vi "TMC.vi"() -> (0 "Position":u32, 1 "Encoder Readout":dbl format="%.3f")   [LabVIEW 2019]
uses:
  TMC Global.vi
panel:
  in  "stop":bool
  in  "Move Up":bool
  out "Soft Down Limit":bool
  out "Soft Up Limit":bool
  out "3.958- Empty Target":bool
  out "2.746 - Carbon Target":bool
  out "1.512 - Bottom Target":bool
  out "0.013 - 10mm Hole":bool
  out "3.200 - Top Target":bool
  out "Moving Down":bool
  out "Moving Up":bool
  in  "Move Down":bool
  out "Boolean":bool
  # "0.040 added by DD/OR 2-15-02"
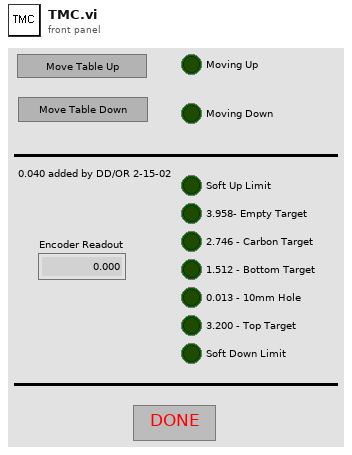
[diagram p1: front panel]
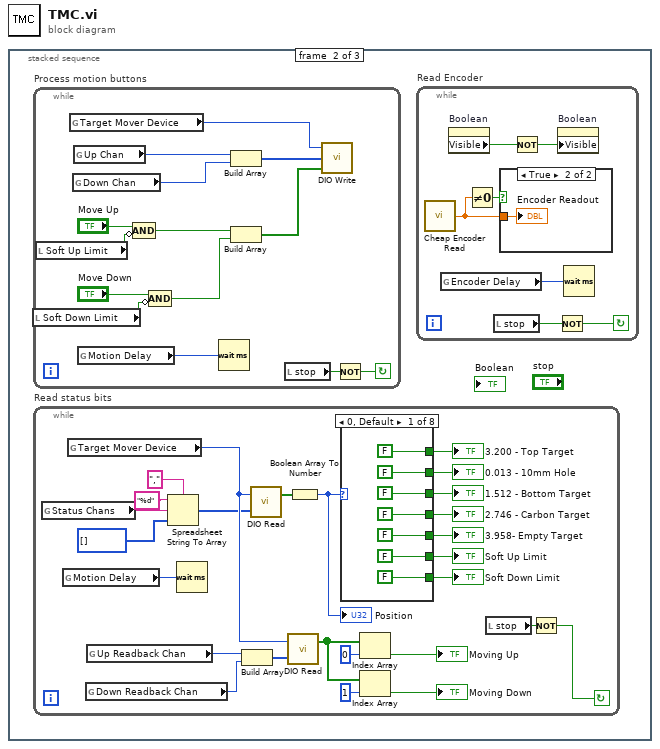
[diagram p0: block diagram]
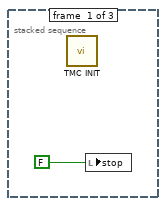
[diagram p2: hidden frame]
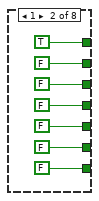
[diagram p3: hidden frame]
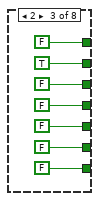
[diagram p4: hidden frame]
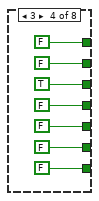
[diagram p5: hidden frame]
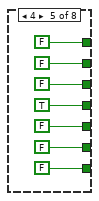
[diagram p6: hidden frame]
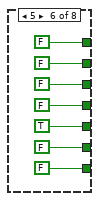
[diagram p7: hidden frame]
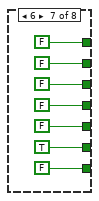
[diagram p8: hidden frame]
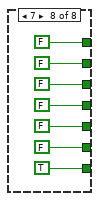
[diagram p9: hidden frame]
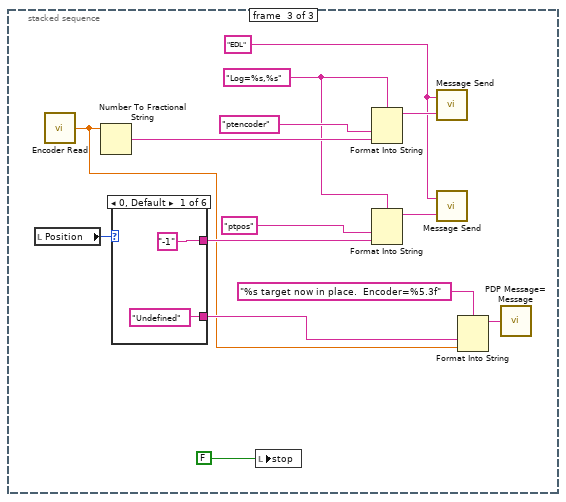
[diagram p11: hidden frame]
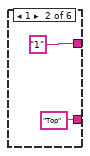
[diagram p12: hidden frame]
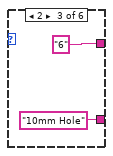
[diagram p13: hidden frame]
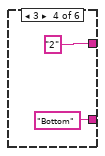
[diagram p14: hidden frame]
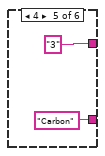
[diagram p15: hidden frame]
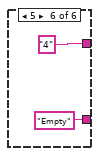
[diagram p16: hidden frame]
diagram:
  n1 = stacked-sequence {
    frame #0 {
      n2 = call "TMC INIT.vi"() -> ()  [unwired: 1 in]
      n3 = local write "stop"(FALSE ("stop")) -> ()
    }
    frame #1 {
      n4 = while "Process motion buttons" {
        stop <- w4 continue-if-true
        n5 = local read "Soft Down Limit"() -> (w8:bool)
        n6 = local read "Soft Up Limit"() -> (w10:bool)
        n7 = global read "TMC Global.vi" "Target Mover Device"() -> (w13:i32)
        n8 = global read "TMC Global.vi" "Down Chan"() -> (w6:i32)
        n9 = global read "TMC Global.vi" "Up Chan"() -> (w15:i32)
        n10 = global read "TMC Global.vi" "Motion Delay"() -> (w12:u32)
        n11 = Compound Arithmetic op=AND("Move Up", invert w10) -> (w2:bool)
        n12 = Compound Arithmetic op=AND("Move Down", invert w8) -> (w3:bool)
        n13 = Wait (ms)(milliseconds to wait=w12) -> ()  [unwired: 1 out]
        n14 = Build Array(w15, w6) -> (w14:i32[])
        n15 = Build Array(w2, w3) -> (w7:bool[])
        n16 = local read "stop"() -> (w5:bool)
        n17 = call "DIO Write.vi"("Data"=w7, "Channels"=w14, "device"=w13) -> ()  [unwired: 1 out]
        n18 = Not(x=w5) -> (.not. x?=w4:bool)
      }
      n19 = while "Read status bits" {
        stop <- w18 continue-if-true
        n20 = global read "TMC Global.vi" "Status Chans"() -> (w38:string)
        n21 = global read "TMC Global.vi" "Motion Delay"() -> (w41:u32)
        n22 = global read "TMC Global.vi" "Target Mover Device"() -> (w23:i32)
        n23 = global read "TMC Global.vi" "Down Readback Chan"() -> (w25:i32)
        n24 = global read "TMC Global.vi" "Up Readback Chan"() -> (w29:i32)
        n25 = Spreadsheet String To Array(delimiter (Tab)=",", format string="%d", spreadsheet string=w38, array type (2D Dbl)=i32[] [] ("Array Constant")) -> (array=w22:i32[])
        n26 = Wait (ms)(milliseconds to wait=w41) -> ()  [unwired: 1 out]
        n27 = Build Array(w29, w25) -> (w28:i32[])
        n28 = call "DIO Read.vi"("Channels"=w22, "device"=w23) -> ("Data"=w21:bool[])  [unwired: 1 out]
        n29 = call "DIO Read.vi"("Channels"=w28, "device"=w23) -> ("Data"=w24:bool[])  [unwired: 1 out]
        n30 = Boolean Array To Number(Boolean array=w21) -> (number=w19:u32)
        "Position" <- w19
        n31 = case shown="0, Default" w19 {
          tunnel: [FALSE TRUE FALSE FALSE FALSE FALSE FALSE FALSE] -> w36
          tunnel: [FALSE FALSE TRUE FALSE FALSE FALSE FALSE FALSE] -> w35
          tunnel: [FALSE FALSE FALSE TRUE FALSE FALSE FALSE FALSE] -> w34
          tunnel: [FALSE FALSE FALSE FALSE TRUE FALSE FALSE FALSE] -> w33
          tunnel: [FALSE FALSE FALSE FALSE FALSE TRUE FALSE FALSE] -> w32
          tunnel: [FALSE FALSE FALSE FALSE FALSE FALSE TRUE FALSE] -> w31
          tunnel: [FALSE FALSE FALSE FALSE FALSE FALSE FALSE TRUE] -> w30
          frame 0, Default {
          }
          frame 1 {
          }
          frame 2 {
          }
          frame 3 {
          }
          frame 4 {
          }
          frame 5 {
          }
          frame 6 {
          }
          frame 7 {
          }
        }
        "Soft Down Limit" <- w30
        "Soft Up Limit" <- w31
        "3.958- Empty Target" <- w32
        "2.746 - Carbon Target" <- w33
        "1.512 - Bottom Target" <- w34
        "0.013 - 10mm Hole" <- w35
        "3.200 - Top Target" <- w36
        n32 = Index Array(array=w24, index=0 ("Index")) -> (element=→"Moving Up":bool)
        n33 = Index Array(array=w24, index=1 ("Index")) -> (element=→"Moving Down":bool)
        n34 = local read "stop"() -> (w20:bool)
        n35 = Not(x=w20) -> (.not. x?=w18:bool)
      }
      n36 = while "Read Encoder" {
        stop <- w100 continue-if-true
        n37 = call "Cheap Encoder Read.vi"() -> ("Encoder Position"=w98:dbl)
        n38 = global read "TMC Global.vi" "Encoder Delay"() -> (w104:u32)
        n39 = property on="Boolean" class="Bool (strict)"() -> ("Visible"=w103:bool)  [unwired: 2 in, 2 out]
        n40 = Not Equal To 0?(x=w98) -> (x != 0?=w99:bool)
        n41 = local read "stop"() -> (w101:bool)
        n42 = case shown="True" w99 {
          tunnel: w98 -> [_ w105]
          frame False {
          }
          frame True {
            "Encoder Readout" <- w105
          }
        }
        n43 = Not(x=w103) -> (.not. x?=w102:bool)
        n44 = Not(x=w101) -> (.not. x?=w100:bool)
        n45 = property on="Boolean" class="Bool (strict)"("Visible"=w102) -> ()  [unwired: 2 in, 2 out]
        n46 = Wait (ms)(milliseconds to wait=w104) -> ()  [unwired: 1 out]
      }
    }
    frame #2 {
      w110 = "EDL"
      w113 = "Log=%s,%s" ("Format String")
      n47 = local read "Position"() -> (w119:u32)
      n48 = call "Encoder Read.vi"() -> ("Encoder Position"=w106:dbl)
      n49 = Number To Fractional String(number=w106) -> (F-format string=w115:string)  [unwired: 3 in]
      n50 = case shown="0, Default" w119 {
        tunnel: ["-1" "1" "6" "2" "3" "4"] -> w117
        tunnel: ["Undefined" "Top" "10mm Hole" "Bottom" "Carbon" "Empty"] -> w107
        frame 0, Default {
        }
        frame 1 {
        }
        frame 2 {
        }
        frame 3 {
        }
        frame 4 {
        }
        frame 5 {
        }
      }
      n51 = local write "stop"(FALSE ("stop")) -> ()
      n52 = Format Into String(format string=w113, "ptencoder" ("Variable Name"), w115) -> (resulting string=w112:string)  [unwired: 2 in, 1 out]
      n53 = Format Into String(format string=w113, "ptpos" ("Variable Name"), w117) -> (resulting string=w111:string)  [unwired: 2 in, 1 out]
      n54 = call "Message Send.vi"("Message"=w112, "Destination"=w110) -> ()
      n55 = call "Message Send.vi"("Message"=w111, "Destination"=w110) -> ()
      n56 = Format Into String(format string="%s target now in place.  Encoder=%5.3f" ("Format String"), w107, w106) -> (resulting string=w109:string)  [unwired: 2 in, 1 out]
      n57 = call "PDP Message= Message.vi"("Message"=w109) -> ()
    }
  }
